vi "BuildPacket.vi"(1 "Data":u8[](array[numeric]), 2 "TxID":u32) -> (0 "MsgTX 2":T1)   [LabVIEW 2017]
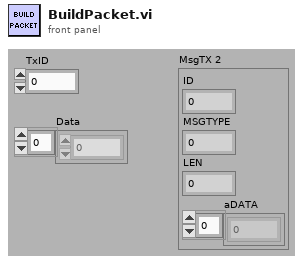
[diagram p1: front panel]
types:
  T1 = cluster{"ID":u32, "MSGTYPE":u8, "LEN":u8, "aDATA":u8[]}
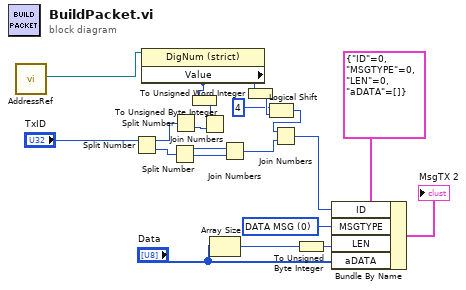
[diagram p0: block diagram]
diagram:
  w20 = u8 0 items=["STATUS"=128, "EXTENDED"=2, "RTR"=1, "DATA MSG"=0] ("MSGTYPE")
  n1 = call "AddressRef.vi"() -> ("add_type out"=w10:refnum<vi>)  [unwired: 11 in]
  n2 = Split Number(x="TxID") -> (hi(x)=w13:u16, lo(x)=w7:u16)
  n3 = property class="DigNum (strict)"(reference=w10) -> ("Value"=w4:u16)  [unwired: 1 in, 2 out]
  n4 = Split Number(x=w7) -> (hi(x)=w11:u8, lo(x)=w12:u8)
  n5 = Split Number(x=w13) -> (lo(x)=w8:u8)  [unwired: 1 out]
  n6 = To Unsigned Byte Integer(number=w4) -> (unsigned 8bit integer=w6:u8)
  n7 = Join Numbers(hi=w6, lo=w8) -> ()  [unwired: 1 out]
  n8 = Array Size(array="Data") -> (size(s)=w15:i32)
  n9 = Join Numbers(hi=w11, lo=w12) -> ((hi.lo)=w9:u16)
  n10 = To Unsigned Word Integer(number=w4) -> (unsigned 16bit integer=w3:u16)
  n11 = Logical Shift(y=i8 4, x=w3) -> (x << y=w1:u16)
  n12 = Join Numbers(hi=w1, lo=w9) -> ((hi.lo)=w5:u32)
  n13 = To Unsigned Byte Integer(number=w15) -> (unsigned 8bit integer=w19:u8)
  n14 = Bundle By Name(cluster=T1 {"ID"=0, "MSGTYPE"=0, "LEN"=0, "aDATA"=[]} ("MsgTX 2"), "ID"=w5, "MSGTYPE"=w20, "LEN"=w19, "aDATA"="Data") -> (→"MsgTX 2":T1)
